vi "Fiducial Scan.vi"(8 "error in":errorcluster, 10 "input cluster":T1, 11 "Gantry In":refnum<k24>) -> (0 "error out":errorcluster, 1 "Not Found?":bool, 2 "output cluster":T1, 3 "Gantry Out":refnum<k24>)   [LabVIEW 2021, in "Component Tray.lvclass"]
uses:
  Component Tray.lvclass
  Find Component.ctl
  Controller/Camera/Machine Vision.ctl
  C:/Program Files (x86)/Aerotech/A3200/LabVIEW/2010/Bin/Aerotech.A3200.dll
  Program Files (x86)/Aerotech/A3200/LabVIEW/2010/Bin/Aerotech.A3200.dll
  Component Tray.lvclass/Component Tray.ctl
  Controller/Motion/A3200/A3200.lvclass
  Controller/Camera/Camera.lvclass
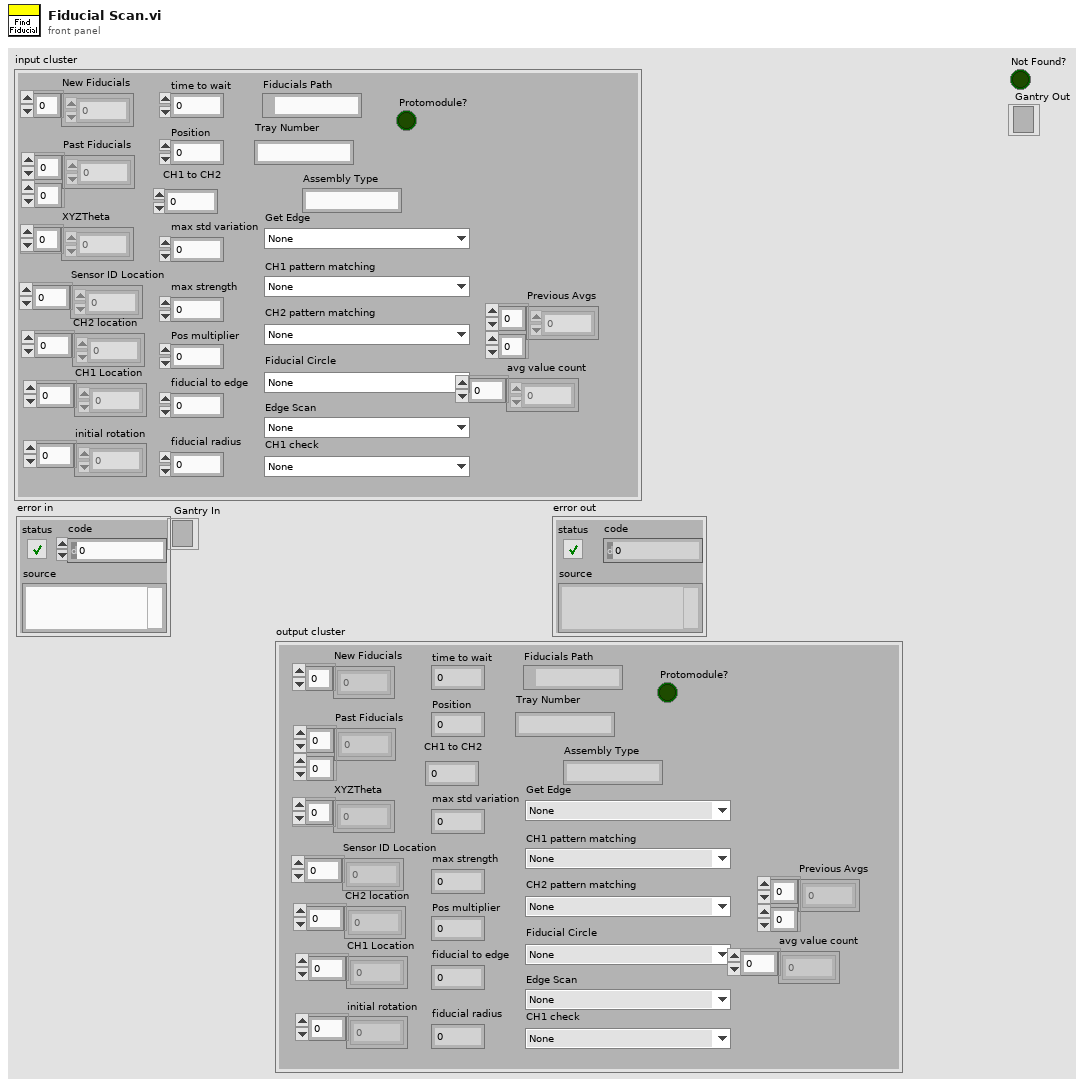
[diagram p1: front panel]
types:
  T1 = typedef "Component Tray.lvclass/Find Component.ctl" = cluster{"New Fiducials":dbl[], "Past Fiducials":dbl[][], "XYZTheta":dbl[], "Fiducials Path":path, "Position":i32, "CH1 Location":dbl[], "Sensor ID Location":dbl[], "initial rotation":dbl[], "CH2 location":dbl[], "max std variation":dbl, "max strength":dbl, "CH2 pattern matching":T2, "Fiducial Circle":T2, "Get Edge":T2, "Pos multiplier":dbl, "time to wait":u32, "fiducial to edge":dbl, "Protomodule?":bool, "Assembly Type":string, "CH1 to CH2":dbl, "Tray Number":string, "fiducial radius":dbl, "4 fiducials?":bool, "CH1 check":T2, "Edge Scan":T2, "CH1 pattern matching":T2, "Sensor Thickness":dbl, "Previous Avgs":dbl[][], "avg value count":dbl[]}
  T2 = typedef "Camera.lvclass/Machine Vision.ctl" = enum16{"None", "Assembly Tray Circle", "Assembly Tray Fiducial", "Partial Hexaboard", "sensor edge init", "HB edge init", "sensor edge pos1", "sensor edge pos2", "HB edge pos1", "HB edge pos2", "Sensor CH1-2", "HB CH1", "HB CH2", "V3 Sensor Circle", "Hexaboard Circle", "sensor CH1 check", "HB CH1 check ", "sensor ID"}
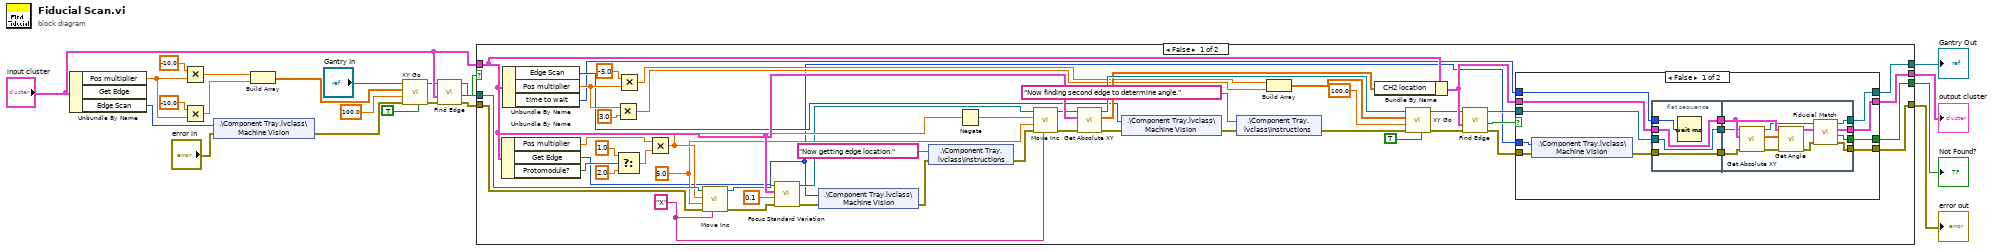
[diagram p0: block diagram]
diagram:
  n1 = Unbundle By Name("input cluster") -> ("Pos multiplier"=w14:dbl, "Edge Scan"=w1:T2)  [unwired: 1 out]
  n2 = Multiply(x=-10.0, y=w14) -> (x*y=w9:dbl)
  n3 = Multiply(x=-10.0, y=w14) -> (x*y=w10:dbl)
  n4 = shared-variable ".\\Component Tray.lvclass\\Machine Vision"(w1, error in="error in") -> (error out=w4:errorcluster)
  n5 = Build Array(w9, w10) -> (w5:dbl[])
  n6 = call "XY Go.vi"("Increment?"=TRUE, "error in (no error)"=w4, "Speed"=100.0, "XY In"=w5, "Gantry In"="Gantry In") -> ("error out"=w2:errorcluster, "Gantry Out"=w3:refnum<k24>)  [unwired: 4 in, 1 out]
  n7 = call "Find Edge.vi"("error in"=w2, "input cluster"="input cluster", "Gantry In"=w3) -> ("error out"=w13:errorcluster, "Error?"=w12:bool, "Gantry Out"=w17:refnum<k24>)  [unwired: 6 in]
  n8 = case shown="False" w12 {
    selector: w12 -> [_ w106]
    tunnel: [w61 w106] -> w22
    tunnel: [w63 w108] -> w21
    tunnel: [w60 w105] -> w20
    tunnel: [w62 w107] -> w19
    tunnel: "input cluster" -> [w70 w107]
    tunnel: w17 -> [w69 w108]
    tunnel: w13 -> [w68 w105]
    frame False {
      w51 = "X" ("Axis")
      w50 = 5.0 ("Speed")
      n9 = Unbundle By Name(w70) -> ("Pos multiplier"=w55:dbl, "Get Edge"=w24:T2, "Protomodule?"=w54:bool)
      n10 = Unbundle By Name(w70) -> ("Edge Scan"=w25:T2, "Pos multiplier"=w59:dbl, "time to wait"=w23:u32)
      n11 = Multiply(x=w59, y=3.0) -> (x*y=w33:dbl)
      n12 = Select(t=1.0 ("y"), s=w54, f=2.0 ("y")) -> (s? t:f=w44:dbl)
      n13 = Multiply(x=-5.0, y=w59) -> (x*y=w37:dbl)
      n14 = Multiply(x=w55, y=w44) -> (x*y=w53:dbl)
      n15 = call "Move Inc.vi"("Axis"=w51, "error in (no error)"=w68, "Speed"=w50, "Distance"=w53, "Gantry In"=w69) -> ("error out"=w48:errorcluster, "Gantry Out"=w47:refnum<k24>)  [unwired: 5 in]
      n16 = call "Focus Standard Variation.vi"("error in"=w48, "Scan Increments"=0.1 ("Scan Inc"), "Component"=w70, "Gantry In"=w47) -> ("error out"=w29:errorcluster, "Gantry Out"=w49:refnum<k24>)  [unwired: 5 in, 1 out]
      n17 = shared-variable ".\\Component Tray.lvclass\\Machine Vision"(w24, error in=w29) -> (error out=w28:errorcluster)
      n18 = shared-variable ".\\Component Tray.lvclass\\Instructions"("Now getting edge location." ("Instructions"), error in=w28) -> (error out=w42:errorcluster)
      n19 = Negate(x=w53) -> (-x=w52:dbl)
      n20 = call "Move Inc.vi"("Axis"=w51, "error in (no error)"=w42, "Speed"=w50, "Distance"=w52, "Gantry In"=w49) -> ("error out"=w56:errorcluster, "Gantry Out"=w57:refnum<k24>)  [unwired: 5 in]
      n21 = call "Get Absolute XY.vi"("error in (no error)"=w56, "Component"=w70, "Gantry In"=w57) -> ("error out"=w27:errorcluster, "Abs XY"=w58:dbl[], "Gantry Out"=w71:refnum<k24>)  [unwired: 6 in]
      n22 = shared-variable ".\\Component Tray.lvclass\\Machine Vision"(w25, error in=w27) -> (error out=w26:errorcluster)
      n23 = shared-variable ".\\Component Tray.lvclass\\Instructions"("Now finding second edge to determine angle." ("Instructions"), error in=w26) -> (error out=w30:errorcluster)
      n24 = Build Array(w37, w33) -> (w38:dbl[])
      n25 = Bundle By Name(cluster=w70, "CH2 location"=w58) -> (w65:T1)
      n26 = call "XY Go.vi"("Increment?"=TRUE, "error in (no error)"=w30, "Speed"=100.0, "XY In"=w38, "Gantry In"=w71) -> ("error out"=w40:errorcluster, "Gantry Out"=w39:refnum<k24>)  [unwired: 4 in, 1 out]
      n27 = call "Find Edge.vi"("error in"=w40, "input cluster"=w65, "Gantry In"=w39) -> ("error out"=w64:errorcluster, "Error?"=w67:bool, "Gantry Out"=w66:refnum<k24>)  [unwired: 6 in]
      n28 = case shown="False" w67 {
        selector: w67 -> [_ w102]
        tunnel: w66 -> [w83 w104]
        tunnel: w65 -> [w84 w103]
        tunnel: w64 -> [w77 w101]
        tunnel: [w82 w104] -> w63
        tunnel: [w81 w103] -> w62
        tunnel: [w80 w102] -> w61
        tunnel: [w79 w101] -> w60
        tunnel: w24 -> [w78 _]
        tunnel: w23 -> [w72 _]
        frame False {
          n29 = shared-variable ".\\Component Tray.lvclass\\Machine Vision"(w78, error in=w77) -> (error out=w76:errorcluster)
          n30 = flat-sequence {
            tunnel: w76 -> [w86]
            tunnel: w83 -> [w87]
            tunnel: w84 -> [w88]
            tunnel: [w88] -> w75
            tunnel: [w87] -> w74
            tunnel: [w86] -> w73
            tunnel: w72 -> [w85]
            tunnel: [w98] -> w82
            tunnel: [w97] -> w81
            tunnel: [w96] -> w80
            tunnel: [w95] -> w79
            tunnel: w75 -> [w100]
            tunnel: w74 -> [w99]
            tunnel: w73 -> [w89]
            frame #0 {
              n31 = Wait (ms)(milliseconds to wait=w85) -> ()  [unwired: 1 out]
            }
            frame #1 {
              n32 = call "Get Absolute XY.vi"("error in (no error)"=w89, "Component"=w100, "Gantry In"=w99) -> ("error out"=w90:errorcluster, "Abs XY"=w91:dbl[], "Gantry Out"=w94:refnum<k24>)  [unwired: 6 in]
              n33 = call "Get Angle.vi"("error in"=w90, "array"=w91, "input cluster"=w100) -> ("error out"=w93:errorcluster, "output cluster"=w92:T1)  [unwired: 7 in]
              n34 = call "Fiducial Match.vi"("error in (no error)"=w93, "input cluster"=w92, "Gantry In"=w94) -> ("error out"=w95:errorcluster, "Not Found?"=w96:bool, "output cluster"=w97:T1, "Gantry Out"=w98:refnum<k24>)  [unwired: 5 in]
            }
          }
        }
        frame True {
        }
      }
    }
    frame True {
    }
  }
  "Not Found?" <- w22
  "error out" <- w20
  "Gantry Out" <- w21
  "output cluster" <- w19
